vi "DCIR.vi"() -> ()   [LabVIEW 2024]
uses:
  <vilib>/Analysis/baseanly.llb/Mean (DBL).vi
  <instrlib>/EFmeter/EFmeter.lvlib
  <vilib>/Analysis/NI_AALBase.lvlib
  <instrlib>/Zatez Kopper/Zatez Kopper.lvlib
  <instrlib>/EFmeter/Examples/BK Precision 8500B Series/BK Precision 8500B Series.lvlib
panel:
  in  "LOAD":refnum<visa-resource-name>
  out "DCIR":dbl
  in  "Èas ustálení [ms]":dbl
  in  "Typ zateze":u16(ring) items=["Manualni", "BK 8542B", "KOPPER-zatez"]
  in  "EFmeter":refnum<visa-resource-name>
  in  "file path (use dialog)":path
  in  "Zatezovaci proud [A]":dbl
  in  "Prumerovani":bool
  in  "Vzorku na krokù":u16 max=100 step=1
  in  "Clear":bool
  in  "Ulozit data":bool
  in  "Start":bool
  in  "stop":bool
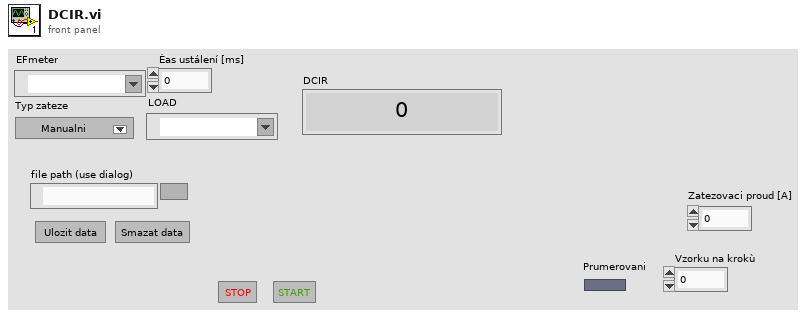
[diagram p1: front panel]
types:
  T1 = enum16{"open", "replace", "create", "open or create", "replace or create", "replace or create with confirmation"}
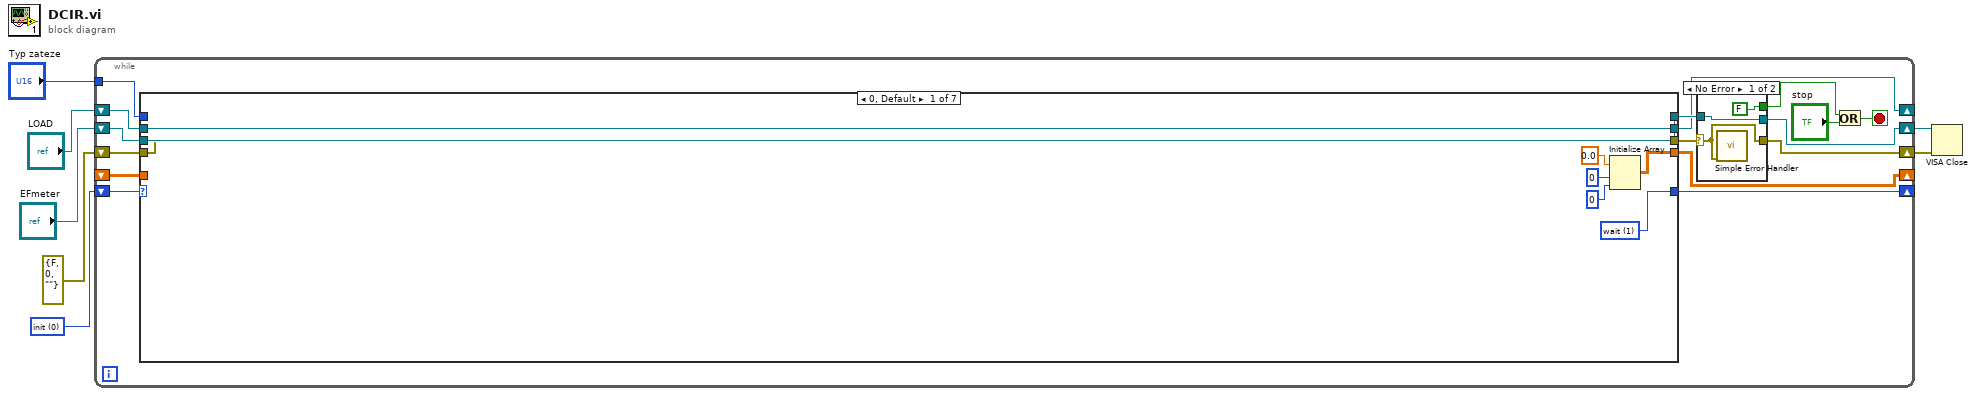
[diagram p0: block diagram]
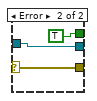
[diagram p2: hidden frame]
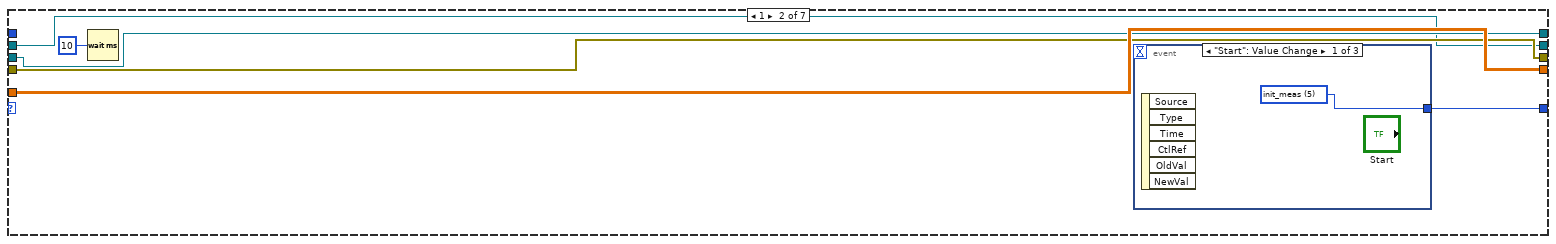
[diagram p3: hidden frame]
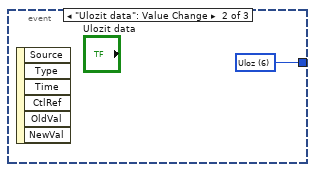
[diagram p4: hidden frame]
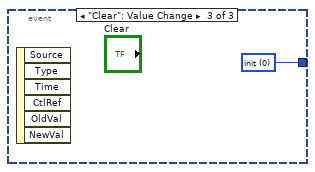
[diagram p5: hidden frame]
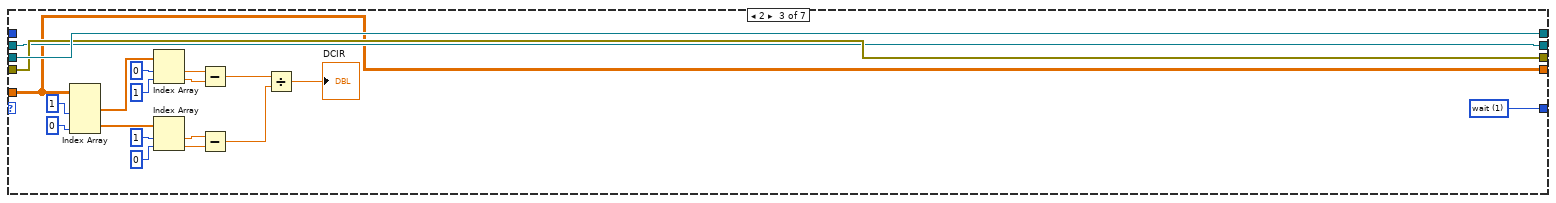
[diagram p6: hidden frame]
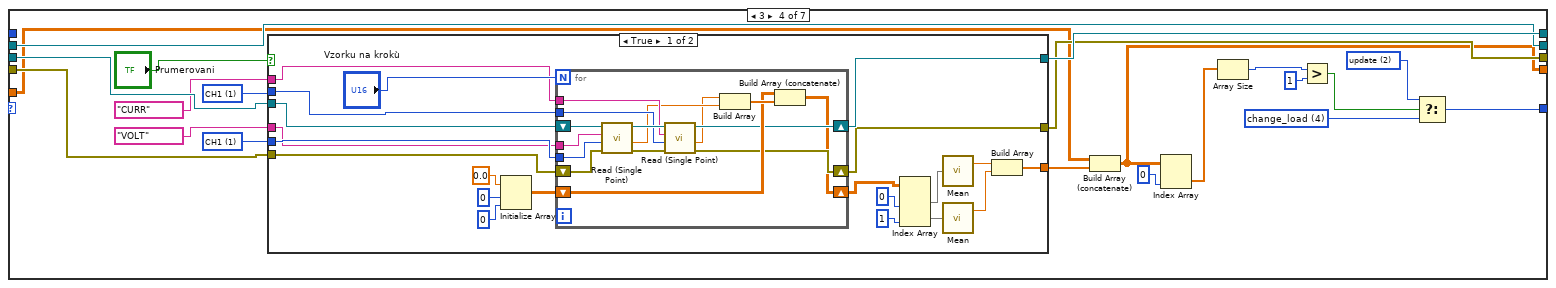
[diagram p7: hidden frame]
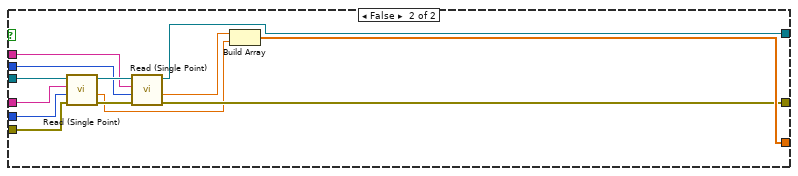
[diagram p8: hidden frame]
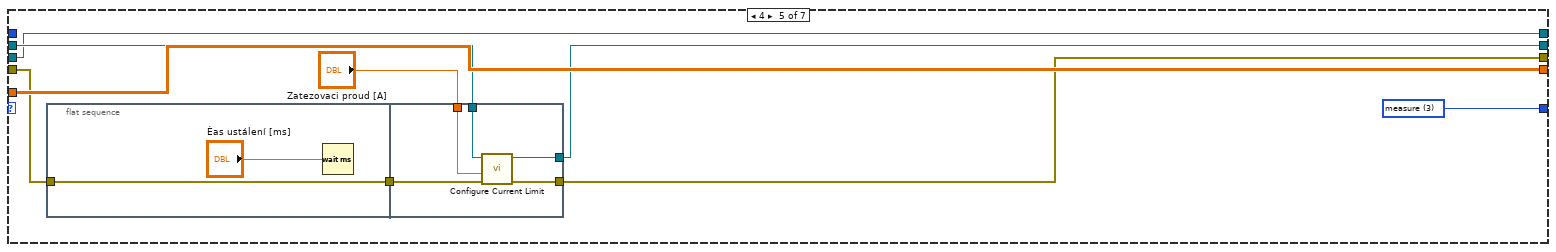
[diagram p9: hidden frame]
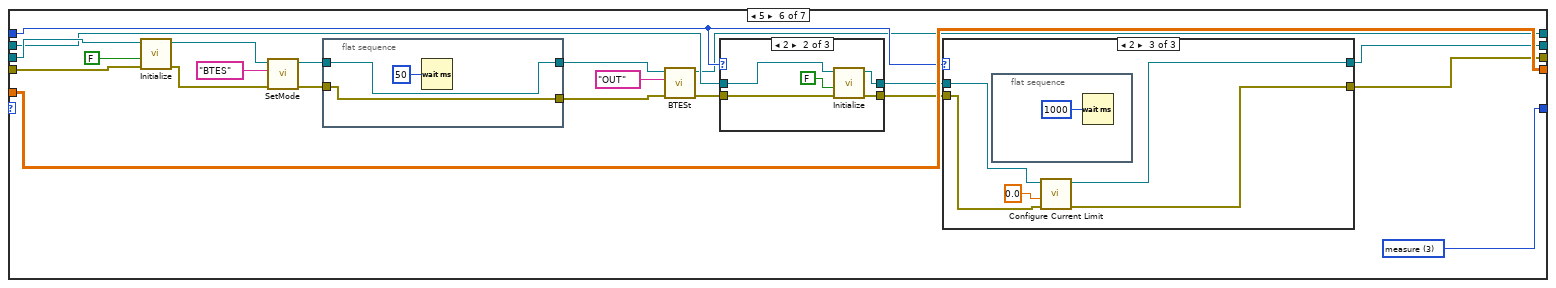
[diagram p10: hidden frame]
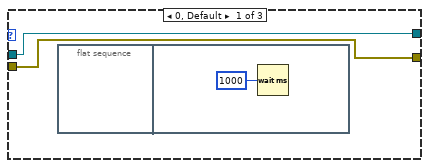
[diagram p11: hidden frame]
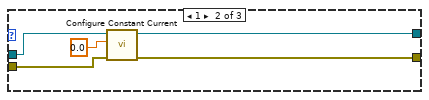
[diagram p12: hidden frame]
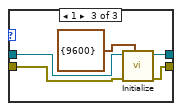
[diagram p14: hidden frame]
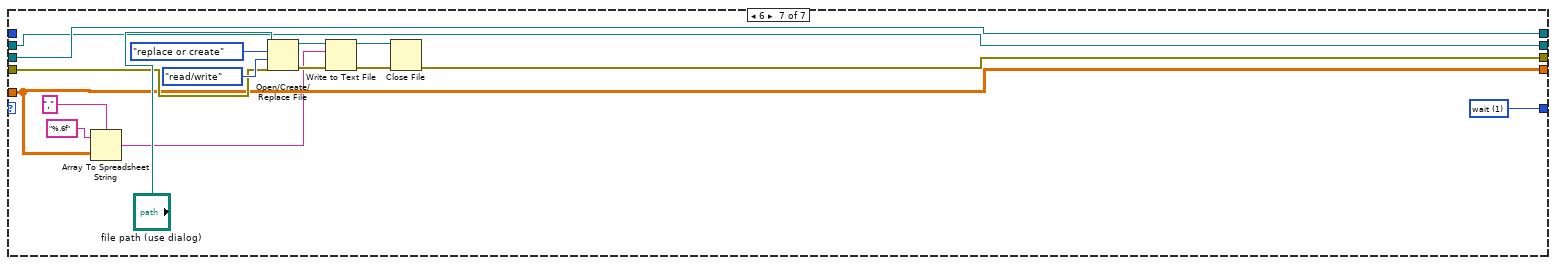
[diagram p15: hidden frame]
diagram:
  w7 = u16 0 items=["init", "wait", "update", "measure", "change_load", "init_meas", "Uloz", "clear"]
  n1 = while {
    shift-right: [w23] -> _
    shift-left: _ -> [w22]
    shift-right: [w18] -> _
    shift-left: w7 -> [w21]
    shift-right: [w15] -> w4
    shift-left: "EFmeter" -> [w20]
    shift-right: [w14] -> w3
    shift-left: errorcluster {"status"=FALSE, "code"=0, "source"=""} ("error in (no error)") -> [w19]
    tunnel: "Typ zateze" -> [w10]
    shift-right: [w9] -> _
    shift-left: "LOAD" -> [w8]
    stop <- w12 stop-if-true
    n2 = case shown="0, Default" w21 {
      tunnel: [w35 w42 w62 w67 w145 w173 w213] -> w23
      tunnel: w22 -> [_ w42 w62 w76 w145 w173 w213]
      tunnel: [w34 w43 w63 w68 w144 w172 w211] -> w18
      tunnel: [w31 w40 w65 w79 w141 w169 w207] -> w17
      tunnel: [w32 w41 w66 w80 w137 w153 w218] -> w16
      tunnel: w20 -> [w32 w41 w66 w86 w137 w165 w218]
      tunnel: w19 -> [w31 w40 w65 w85 w142 w166 w214]
      tunnel: w10 -> [_ _ _ _ _ w167 _]
      tunnel: [w30 w38 w64 w77 w138 w168 w203] -> w9
      tunnel: w8 -> [w30 w38 w64 w77 w139 w155 w203]
      frame 0, Default {
        w34 = u16 1 items=["init", "wait", "update", "measure"]
        n3 = Initialize Array(0.0 ("element"), 0 ("dimension size"), 0 ("dimension size")) -> (w35:dbl[][])
      }
      frame 1 {
        n4 = Wait (ms)(milliseconds to wait=u32 10) -> ()  [unwired: 1 out]
        n5 = event shown="[0] \"Start\": Value Change" {
          selector: _ -> [_ _ _]
          dyn-events: _ -> [_ _ _]
          timeout: _ -> [_ _ _]
          tunnel: [w44 w45 w46] -> w43
          event "Start": Value Change {
            w44 = u16 5 items=["init", "wait", "update", "measure", "change_load", "init_meas"]
            n6 = event-data() -> ()  [unwired: 1 in, 6 out]
          }
          event "Ulozit data": Value Change {
            w45 = u16 6 items=["init", "wait", "update", "measure", "change_load", "init_meas", "Uloz"]
            n7 = event-data() -> ()  [unwired: 1 in, 6 out]
          }
          event "Clear": Value Change {
            w46 = u16 0 items=["init", "wait", "update", "measure", "change_load", "init_meas", "Uloz", "clear"]
            n8 = event-data() -> ()  [unwired: 1 in, 6 out]
          }
        }
      }
      frame 2 {
        w63 = u16 1 items=["init", "wait", "update", "measure", "change_load", "init_meas"]
        n9 = Index Array(array=w62, index (col) #1=1 ("disabled index (col)"), index (col) #2=0 ("index (col)")) -> (element #1=w59:dbl[], element #2=w54:dbl[])  [unwired: 2 in]
        n10 = Index Array(array=w59, index #1=0 ("index"), index #2=1 ("index")) -> (element #1=w56:dbl, element #2=w55:dbl)
        n11 = Index Array(array=w54, index #1=1 ("index"), index #2=0 ("index")) -> (element #1=w51:dbl, element #2=w50:dbl)
        n12 = Subtract(x=w56, y=w55) -> (x-y=w48:dbl)
        n13 = Subtract(x=w51, y=w50) -> (x-y=w49:dbl)
        n14 = Divide(x=w48, y=w49) -> (x/y=→"DCIR":dbl)
      }
      frame 3 {
        w70 = u16 4 items=["init", "wait", "update", "measure", "change_load", "init_meas", "Uloz", "clear"]
        w81 = u16 1 items=["CH2"=2, "CH1"=1] ("Ring")
        w84 = u16 1 items=["CH2"=2, "CH1"=1] ("Ring")
        w69 = u16 2 items=["init", "wait", "update", "measure"]
        n15 = case shown="True" "Prumerovani" {
          tunnel: [w90 w136] -> w87
          tunnel: w86 -> [w103 w135]
          tunnel: w85 -> [w102 w134]
          tunnel: w84 -> [w101 w133]
          tunnel: "VOLT" ("Combo Box") -> [w100 w132]
          tunnel: "CURR" ("Combo Box") -> [w99 w129]
          tunnel: w81 -> [w98 w128]
          tunnel: [w89 w127] -> w80
          tunnel: [w88 w126] -> w79
          frame True {
            n16 = Initialize Array(0.0 ("element"), 0 ("dimension size"), 0 ("dimension size")) -> (w104:dbl[][])
            n17 = for {
              N: "Vzorku na krokù" -> [_]
              shift-right: [w118] -> w89
              shift-left: w103 -> [w119]
              shift-right: [w116] -> w88
              shift-left: w102 -> [w117]
              tunnel: w101 -> [w115]
              tunnel: w100 -> [w114]
              tunnel: w99 -> [w113]
              tunnel: w98 -> [w112]
              shift-right: [w111] -> w97
              shift-left: w104 -> [w120]
              n18 = call <instrlib>:"Read (Single Point).vi"("error in (no error)"=w117, "Ring"=w115, "Combo Box"=w114, "VISA resource name"=w119) -> ("error out"=w122:errorcluster, "Measurement"=w110:dbl, "VISA resource name out"=w123:refnum<visa-resource-name>)  [unwired: 5 in]
              n19 = call <instrlib>:"Read (Single Point).vi"("error in (no error)"=w122, "Ring"=w112, "Combo Box"=w113, "VISA resource name"=w123) -> ("error out"=w116:errorcluster, "Measurement"=w109:dbl, "VISA resource name out"=w118:refnum<visa-resource-name>)  [unwired: 5 in]
              n20 = Build Array(w109, w110) -> (w121:dbl[])
              n21 = Build Array (concatenate)(w120, w121) -> (w111:dbl[][])
            }
            n22 = Index Array(array=w97, index (col) #1=0 ("disabled index (col)"), index (col) #2=1 ("index (col)")) -> (element #1=w96:dbl[], element #2=w95:dbl[])  [unwired: 2 in]
            n23 = call-poly <vilib>:"Mean.vi"("X"=w96) -> ("mean"=w92:dbl)  [unwired: 1 out]
            n24 = call-poly <vilib>:"Mean.vi"("X"=w95) -> ("mean"=w91:dbl)  [unwired: 1 out]
            n25 = Build Array(w92, w91) -> (w90:dbl[])
          }
          frame False {
            n26 = call <instrlib>:"Read (Single Point).vi"("error in (no error)"=w134, "Ring"=w133, "Combo Box"=w132, "VISA resource name"=w135) -> ("error out"=w131:errorcluster, "Measurement"=w125:dbl, "VISA resource name out"=w130:refnum<visa-resource-name>)  [unwired: 5 in]
            n27 = call <instrlib>:"Read (Single Point).vi"("error in (no error)"=w131, "Ring"=w128, "Combo Box"=w129, "VISA resource name"=w130) -> ("error out"=w126:errorcluster, "Measurement"=w124:dbl, "VISA resource name out"=w127:refnum<visa-resource-name>)  [unwired: 5 in]
            n28 = Build Array(w124, w125) -> (w136:dbl[])
          }
        }
        n29 = Build Array (concatenate)(w76, w87) -> (w67:dbl[][])
        n30 = Index Array(array=w67, index (col)=0 ("disabled index (col)")) -> (element=w74:dbl[])  [unwired: 1 in]
        n31 = Array Size(array=w74) -> (size(s)=w73:i32)
        n32 = Greater?(x=w73, y=1) -> (0:w71:bool)
        n33 = Select(t=w69, s=w71, f=w70) -> (s? t:f=w68:u16)
      }
      frame 4 {
        w144 = u16 3 items=["init", "wait", "update", "measure", "change_load", "init_meas", "Uloz", "clear"]
        n34 = flat-sequence {
          tunnel: w142 -> [w146]
          tunnel: [w146] -> w143
          tunnel: w143 -> [w152]
          tunnel: [w151] -> w141
          tunnel: [w150] -> w138
          tunnel: "Zatezovaci proud [A]" -> [w149]
          tunnel: w139 -> [w148]
          frame #0 {
            n35 = Wait (ms)(milliseconds to wait="Èas ustálení [ms]") -> ()  [unwired: 1 out]
          }
          frame #1 {
            n36 = call <instrlib>:"Configure Current Limit.vi"("error in (no error)"=w152, "Current Limit (0.0 A)"=w149, "VISA resource name"=w148) -> ("error out"=w151:errorcluster, "VISA resource name out"=w150:refnum<visa-resource-name>)  [unwired: 7 in]
          }
        }
      }
      frame 5 {
        w172 = u16 3 items=["init", "wait", "update", "measure", "change_load", "init_meas"]
        n37 = call <instrlib>:"Initialize.vi"("error in (no error)"=w166, "Reset (True)"=FALSE, "VISA resource name"=w165) -> ("error out"=w161:errorcluster, "VISA resource name out"=w163:refnum<visa-resource-name>)  [unwired: 7 in]
        n38 = call <instrlib>:"SetMode.vi"("error in (no error)"=w161, "Combo Box"="BTES", "VISA resource name"=w163) -> ("error out"=w160:errorcluster, "VISA resource name out"=w159:refnum<visa-resource-name>)  [unwired: 7 in]
        n39 = flat-sequence {
          tunnel: [w200] -> w154
          tunnel: [w201] -> w158
          tunnel: w160 -> [w201]
          tunnel: w159 -> [w200]
          frame #0 {
            n40 = Wait (ms)(milliseconds to wait=u32 50) -> ()  [unwired: 1 out]
          }
        }
        n41 = call <instrlib>:"BTESt.vi"("error in (no error)"=w158, "Combo Box"="OUT", "VISA resource name"=w154) -> ("error out"=w156:errorcluster, "VISA resource name out"=w153:refnum<visa-resource-name>)  [unwired: 7 in]
        n42 = case shown="2" w167 {
          tunnel: w156 -> [w189 w193 w198]
          tunnel: [w189 w192 w197] -> w171
          tunnel: [w188 w191 w196] -> w170
          tunnel: w155 -> [w188 w194 w195]
          frame 0, Default {
          }
          frame 2 {
            n43 = call <instrlib>:"Initialize.vi"("error in (no error)"=w193, "Reset (True)"=FALSE, "VISA resource name"=w194) -> ("error out"=w192:errorcluster, "VISA resource name out"=w191:refnum<visa-resource-name>)  [unwired: 7 in]
          }
          frame 1 {
            n44 = call <instrlib>:"Initialize.vi"("Serial Configuration"=cluster{"Baud Rate":u32} {"Baud Rate"=9600}, "error in (no error)"=w198, "VISA resource name"=w195) -> ("error out"=w197:errorcluster, "VISA resource name out"=w196:refnum<visa-resource-name>)  [unwired: 7 in]
          }
        }
        n45 = case shown="2" w167 {
          tunnel: w170 -> [w175 w181 w183]
          tunnel: [w175 w180 w186] -> w168
          tunnel: w171 -> [w174 w179 w184]
          tunnel: [w174 w178 w185] -> w169
          frame 0, Default {
            n46 = flat-sequence {
              frame #0 {
              }
              frame #1 {
                n47 = Wait (ms)(milliseconds to wait=u32 1000) -> ()  [unwired: 1 out]
              }
            }
          }
          frame 1 {
            n48 = call <instrlib>:"Configure Constant Current.vi"("error in (no error)"=w179, "CC Current (0)"=0.0, "VISA resource name"=w181) -> ("error out"=w178:errorcluster, "VISA resource name out"=w180:refnum<visa-resource-name>)  [unwired: 7 in]
          }
          frame 2 {
            n49 = flat-sequence {
              frame #0 {
                n50 = Wait (ms)(milliseconds to wait=u32 1000) -> ()  [unwired: 1 out]
              }
            }
            n51 = call <instrlib>:"Configure Current Limit.vi"("error in (no error)"=w184, "Current Limit (0.0 A)"=0.0, "VISA resource name"=w183) -> ("error out"=w185:errorcluster, "VISA resource name out"=w186:refnum<visa-resource-name>)  [unwired: 7 in]
          }
        }
      }
      frame 6 {
        w211 = u16 1 items=["init", "wait", "update", "measure", "change_load", "init_meas"]
        n52 = Array To Spreadsheet String(delimiter (Tab)=",", array=w213, 3:"%.6f" ("format string")) -> (spreadsheet string=w204:string)
        n53 = Open/Create/Replace File(file path (use dialog)="file path (use dialog)", error in=w214, operation (0:open)=T1."replace or create", access (0:read/write)=enum16{"read/write", "read-only", "write-only"}."read/write") -> (refnum out=w206:refnum<file>, error out=w209:errorcluster)  [unwired: 2 in, 1 out]
        n54 = Write to Text File(file (use dialog)=w206, text=w204, error in=w209) -> (refnum out=w205:refnum<file>, error out=w208:errorcluster)  [unwired: 1 in, 1 out]
        n55 = Close File(refnum=w205, error in=w208) -> (error out=w207:errorcluster)  [unwired: 1 out]
      }
    }
    n56 = case shown="No Error" w17 {
      selector: w17 -> [w24 w28]
      tunnel: w16 -> [w26 w29]
      tunnel: [w26 w29] -> w15
      tunnel: [w24 w28] -> w14
      tunnel: [FALSE TRUE] -> w11
      frame No Error {
        n57 = call <vilib>:"Simple Error Handler.vi"("error in (no error)"=w24) -> ()  [unwired: 4 in, 5 out]
      }
      frame Error {
      }
    }
    n58 = Or(x=w11, y="stop") -> (x .or. y?=w12:bool)
  }
  n59 = VISA Close(VISA resource name=w4, error in (no error)=w3) -> ()  [unwired: 1 out]
